vi "niRFUtil WFM Moving Average (real array).vi"(0 "Array In":T1 min=0 max=127 format="%.2f", 5 "Averaging Window (samples)":i32=20) -> (4 "Averaged Array Out":T1 min=0 max=127 format="%.2f")   [LabVIEW 2015, in "niRFUtil.lvlib"]
uses:
  niRFUtil.lvlib
  Includes/niRFUtil INC Real Array.ctl
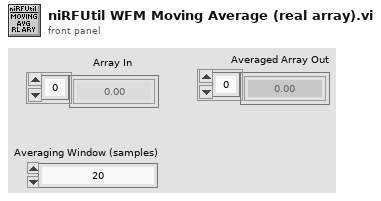
[diagram p1: front panel]
types:
  T1 = typedef "niRFUtil.lvlib/niRFUtil INC Real Array.ctl" = sgl[]
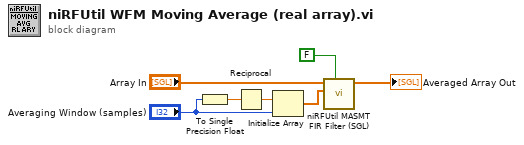
[diagram p0: block diagram]
diagram:
  n1 = To Single Precision Float(number="Averaging Window (samples)") -> (single precision float=w6:sgl)
  n2 = Reciprocal(x=w6) -> (1/x=w7:sgl)
  n3 = Initialize Array(w7, "Averaging Window (samples)") -> (w2:sgl[])
  n4 = call "niRFUtil MASMT FIR Filter (SGL).vi"("continue?"=FALSE, "FIR Coefficients"=w2, "X"="Array In") -> ("Filtered X"=→"Averaged Array Out":sgl[])  [unwired: 7 in, 1 out]
